vi "report data.vi"() -> (0 "Model Selection":i32, 1 "VW_ Medium":T1, 3 "SK Global":T1, 6 "Data":string[](array[string]))   [LabVIEW 2015]
uses:
  Galobal variable_TI.vi
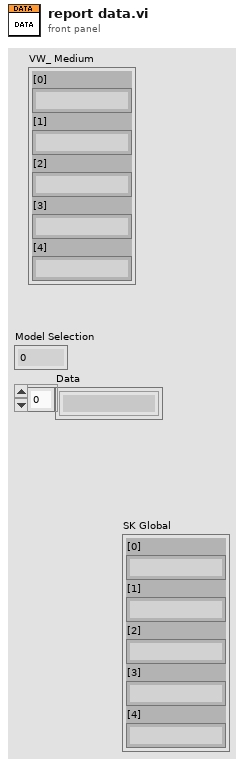
[diagram p1: front panel]
types:
  T1 = cluster{"[0]":string, "[1]":string, "[2]":string, "[3]":string, "[4]":string}
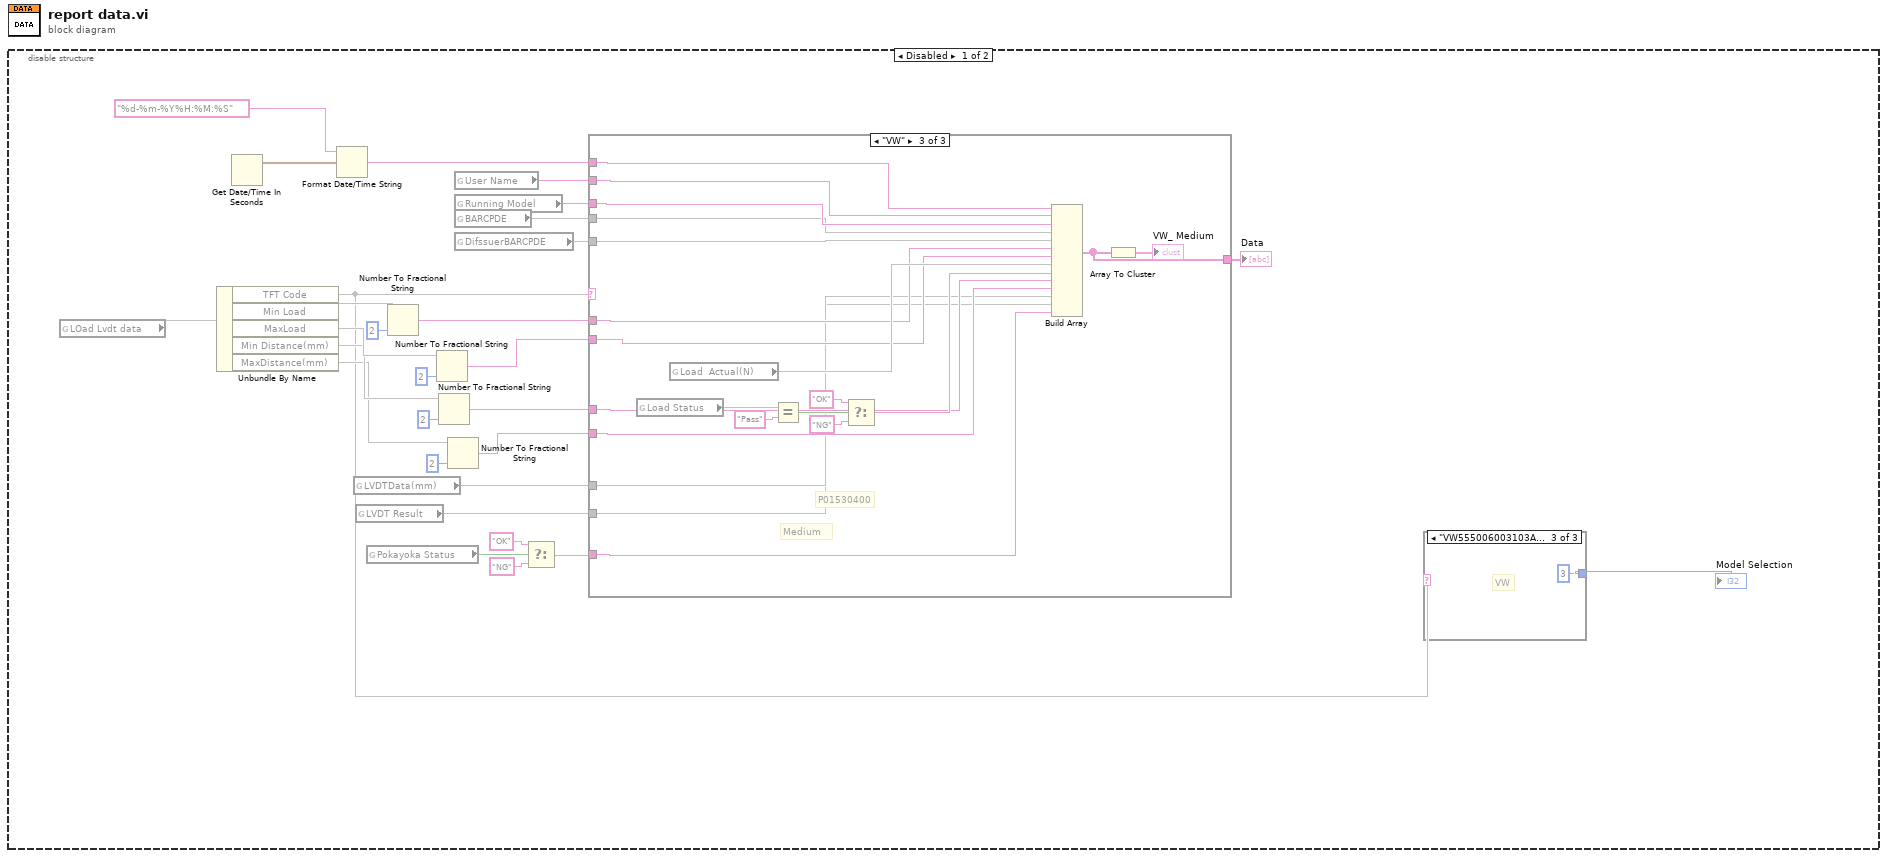
[diagram p0: block diagram]
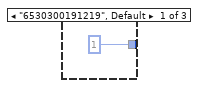
[diagram p2: hidden frame]
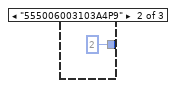
[diagram p3: hidden frame]
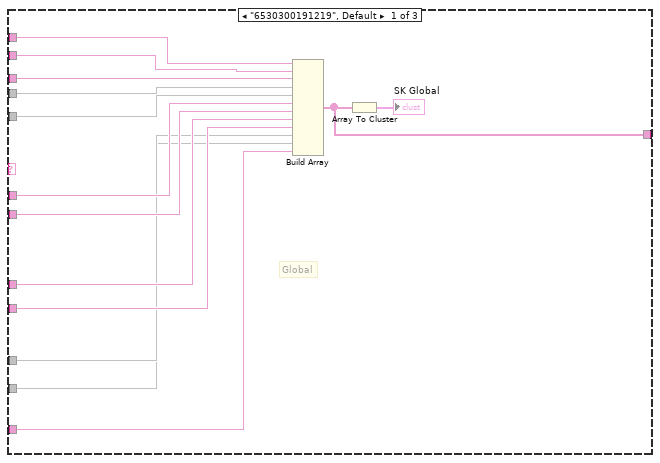
[diagram p4: hidden frame]
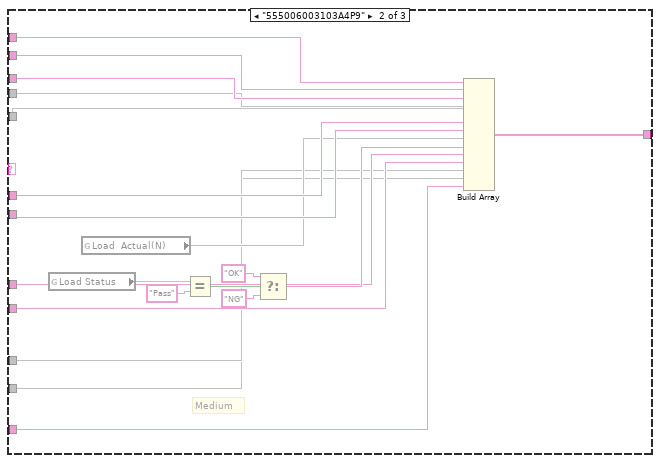
[diagram p5: hidden frame]
diagram:
  n1 = disable-structure shown="Disabled" {
    frame Disabled {
      n2 = global read "Galobal variable_TI.vi" "LOad Lvdt data"() -> (w29)
      n3 = Unbundle By Name(w29) -> ("TFT Code"=w3, "Min Load"=w28, "MaxLoad"=w23, "Min Distance(mm)"=w22, "MaxDistance(mm)"=w21)
      n4 = Get Date/Time In Seconds() -> (seconds since 1Jan1904=w8:timestamp)
      n5 = Format Date/Time String(time format string (%c)="%d-%m-%Y%H:%M:%S", seconds (now)=w8) -> (date/time string=w7:string)  [unwired: 1 in]
      n6 = global read "Galobal variable_TI.vi" "LVDTData(mm)"() -> (w4)
      n7 = global read "Galobal variable_TI.vi" "LVDT Result"() -> (w5)
      n8 = global read "Galobal variable_TI.vi" "Pokayoka Status"() -> (w14:bool)
      n9 = Number To Fractional String(number=w28, precision (6)=i16 2) -> (F-format string=w20:string)  [unwired: 2 in]
      n10 = Number To Fractional String(number=w23, precision (6)=i16 2) -> (F-format string=w19:string)  [unwired: 2 in]
      n11 = Number To Fractional String(number=w22, precision (6)=i16 2) -> (F-format string=w18:string)  [unwired: 2 in]
      n12 = Number To Fractional String(number=w21, precision (6)=i16 2) -> (F-format string=w17:string)  [unwired: 2 in]
      n13 = global read "Galobal variable_TI.vi" "User Name"() -> (w12:string)
      n14 = global read "Galobal variable_TI.vi" "Running Model"() -> (w11:string)
      n15 = global read "Galobal variable_TI.vi" "BARCPDE"() -> (w10)
      n16 = global read "Galobal variable_TI.vi" "DifssuerBARCPDE"() -> (w9)
      n17 = Select(t="OK", s=w14, f="NG") -> (s? t:f=w13:string)
      n18 = case shown="\"VW\"" w3 {
        tunnel: w20 -> [w41 w66 w74]
        tunnel: w19 -> [w40 w65 w73]
        tunnel: w18 -> [w39 w57 w72]
        tunnel: w17 -> [w38 w56 w71]
        tunnel: w13 -> [w35 w55 w68]
        tunnel: w12 -> [w45 w54 w78]
        tunnel: w11 -> [w44 w53 w77]
        tunnel: w10 -> [w43 w52 w76]
        tunnel: w9 -> [w42 w51 w75]
        tunnel: w7 -> [w46 w50 w79]
        tunnel: w5 -> [w36 w48 w69]
        tunnel: w4 -> [w37 w49 w70]
        tunnel: [w33 w47 w67] -> w1
        frame "6530300191219", Default {
          # "Global"
          n19 = Build Array(w46, w45, w44, w43, w42, w41, w40, w39, w38, w37, w36, w35) -> (w33:string[])
          n20 = Array To Cluster(array=w33) -> (cluster=→"SK Global":T1)
        }
        frame "555006003103A4P9" {
          # "Medium"
          n21 = global read "Galobal variable_TI.vi" "Load Status"() -> (w63)
          n22 = global read "Galobal variable_TI.vi" "Load  Actual(N)"() -> (w64)
          n23 = Equal?(x=w63, y="Pass") -> (x = y?=w61:bool)
          n24 = Select(t="OK", s=w61, f="NG") -> (s? t:f=w58:string)
          n25 = Build Array(w50, w54, w53, w52, w51, w66, w65, w64, w58, w57, w56, w49, w48, w55) -> (w47:string[])
        }
        frame "VW" {
          # "Medium"
          # "P01530400"
          n26 = global read "Galobal variable_TI.vi" "Load Status"() -> (w86)
          n27 = global read "Galobal variable_TI.vi" "Load  Actual(N)"() -> (w87)
          n28 = Equal?(x=w86, y="Pass") -> (x = y?=w84:bool)
          n29 = Select(t="OK", s=w84, f="NG") -> (s? t:f=w81:string)
          n30 = Build Array(w79, w78, w77, w76, w75, w74, w73, w87, w81, w72, w71, w70, w69, w68) -> (w67:string[])
          n31 = Array To Cluster(array=w67) -> (cluster=→"VW_ Medium":T1)
        }
      }
      "Data" <- w1
      n32 = case shown="\"VW555006003103A4P9\"" w3 {
        tunnel: [1 2 3] -> w2
        frame "6530300191219", Default {
        }
        frame "555006003103A4P9" {
        }
        frame "VW555006003103A4P9" {
          # "VW"
        }
      }
      "Model Selection" <- w2
    }
    frame Enabled {
    }
  }
